vi "Load Config.vi"(8 "error in (no error)":errorcluster, 11 "Volatus Core in":refnum<class "Volatus Core.lvclass">) -> (0 "error out":errorcluster, 3 "Volatus Core out":refnum<class "Volatus Core.lvclass">, 4 "Validation Errors":errorcluster)   [LabVIEW 2023, in "Volatus.lvlib" / "Volatus Core.lvclass"]
uses:
  Volatus Core.lvclass
  Volatus Core.lvclass/Volatus Core.ctl
  lv-vecto/Vecto/Node Config/Node Config.lvclass/Node Config.ctl
  Module/Module.lvclass/Module.ctl
  VolatusConfig/Node/Node Config.lvclass
  VolatusConfig/VolatusConfig/VolatusConfig.lvclass
  VolatusConfig/VolatusConfig.lvlib
  Module/Module.lvclass
  lv-vecto/Vecto/Node Config/Node Config.lvclass
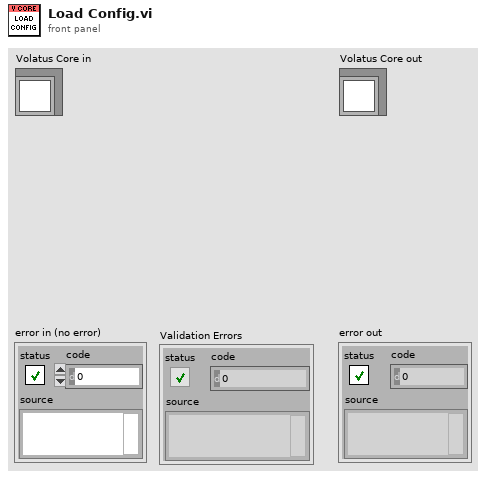
[diagram p1: front panel]
types:
  T1 = typedef "Volatus.lvlib/Volatus Core.lvclass/Config Type.ctl" = enum16{"App INI", "Memory", "Unconfigured"}
  T2 = typedef "VolatusConfig.lvlib/Config Format.ctl" = enum16{"JSON", "INI", "SQLite"}
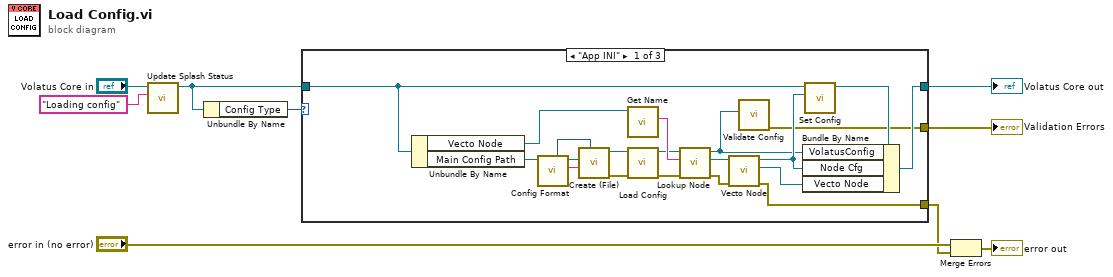
[diagram p0: block diagram]
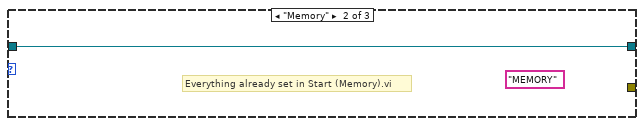
[diagram p2: hidden frame]
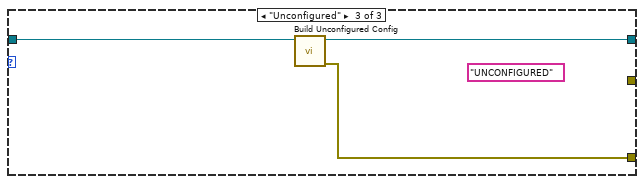
[diagram p3: hidden frame]
diagram:
  n1 = call "Update Splash Status.vi"("Status"="Loading config", "Volatus Core in"="Volatus Core in") -> ("Volatus Core out"=w3:refnum<class "Volatus Core.lvclass">)  [unwired: 8 in, 1 out]
  n2 = Unbundle By Name(w3) -> ("Config Type"=w6:T1)
  n3 = case shown="\"App INI\"" w6 {
    tunnel: [w25 w30 w32] -> w4
    tunnel: [w18 _ w31] -> w5
    tunnel: w3 -> [w22 w30 w33]
    tunnel: [w10 _ _] -> w1
    frame "App INI" {
      n4 = Unbundle By Name(w22) -> ("Vecto Node"=w29:refnum<class "Node Config.lvclass">, "Main Config Path"=w15:path)
      n5 = call "Config Format.vi"("Config Path"=w15) -> ("filename without extension"=w13:string, "Folder"=w14:path, "Format"=w12:T2)  [unwired: 8 in]
      n6 = call "Create (File).vi"("Main Format"=w12, "Main Filename"=w13, "Config Root"=w14) -> ("error out"=w27:errorcluster, "VolatusConfig out"=w28:refnum<class "VolatusConfig.lvclass">)  [unwired: 7 in]
      n7 = call "Get Name.vi"("Node in"=w29) -> ("Name"=w26:string)  [unwired: 8 in, 2 out]
      n8 = call "Load Config.vi"("error in (no error)"=w27, "VolatusConfig in"=w28) -> ("error out"=w16:errorcluster, "VolatusConfig out"=w17:refnum<class "VolatusConfig.lvclass">)  [unwired: 7 in, 1 out]
      n9 = call "Lookup Node.vi"("error in (no error)"=w16, "Node Name"=w26, "VolatusConfig in"=w17) -> ("error out"=w19:errorcluster, "Node"=w23:refnum<class "Node Config.lvclass">, "VolatusConfig out"=w11:refnum<class "VolatusConfig.lvclass">)  [unwired: 6 in]
      n10 = call "Vecto Node.vi"("error in (no error)"=w19, "Node in"=w23) -> ("error out"=w18:errorcluster, "Vecto Node"=w20:refnum<class "Node Config.lvclass">, "Node out"=w21:refnum<class "Node Config.lvclass">)  [unwired: 7 in]
      n11 = call "Validate Config.vi"("VolatusConfig"=w11) -> ("error out"=w10:errorcluster)  [unwired: 10 in]
      n12 = call "Set Config.vi"("Config"=w21, "Module in"=w22) -> ("Module out"=w24:refnum<class "Volatus Core.lvclass">)  [unwired: 9 in]
      n13 = Bundle By Name(cluster=w24, "VolatusConfig"=w11, "Node Cfg"=w21, "Vecto Node"=w20) -> (w25:refnum<class "Volatus Core.lvclass">)
    }
    frame "Memory" {
      (unwired) "MEMORY"
      # "Everything already set in Start (Memory).vi"
    }
    frame "Unconfigured" {
      (unwired) "UNCONFIGURED"
      n14 = call "Build Unconfigured Config.vi"("Volatus Core in"=w33) -> ("error out"=w31:errorcluster, "Volatus Core out"=w32:refnum<class "Volatus Core.lvclass">)  [unwired: 9 in]
    }
  }
  "Volatus Core out" <- w4
  "Validation Errors" <- w1
  n15 = Merge Errors("error in (no error)", w5) -> (→"error out":errorcluster)
